vi "Read Digital Voltmeter.vi"(8 "error in (no error)":errorcluster, 11 "VISA resource name":refnum<visa-resource-name>) -> (0 "error out":errorcluster, 1 "5-digit Frequency":dbl, 2 "3-digit DVM":dbl, 3 "VISA resource name out":refnum<visa-resource-name>)   [LabVIEW 2017, in "Agilent 2000 3000 X-Series.lvlib"]
doc: "Returns the displayed value of the digital voltmeter (DVM)."
uses:
  Agilent 2000 3000 X-Series.lvlib
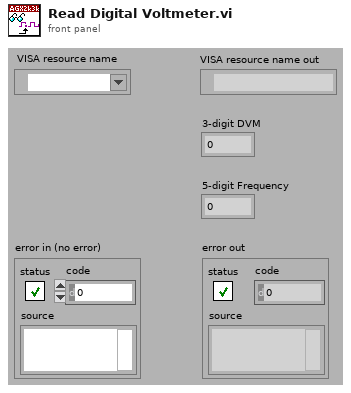
[diagram p1: front panel]
types:
  T1 = typedef "Agilent 2000 3000 X-Series.lvlib/Extended User Data.ctl" = cluster{"X-Series Mode":u16, "Acquisition Type (0: Normal)":i32}
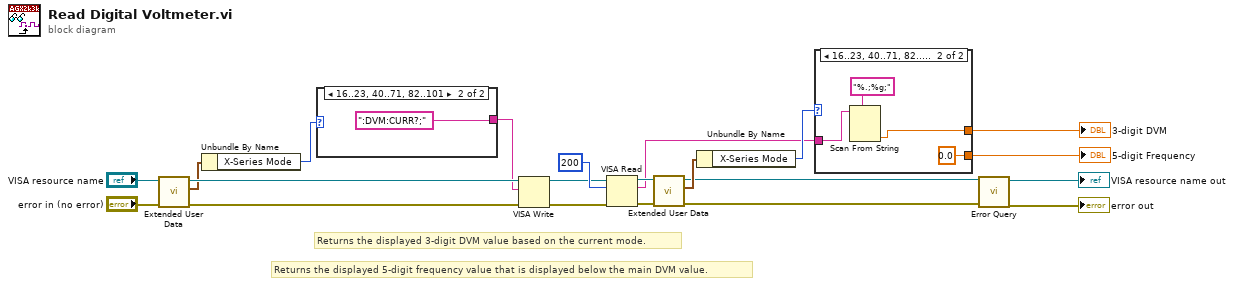
[diagram p0: block diagram]
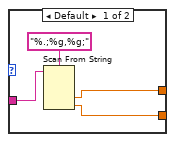
[diagram p2: hidden frame]
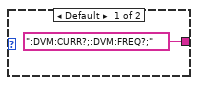
[diagram p3: hidden frame]
diagram:
  # "Returns the displayed 5-digit frequency value that is displayed below the main DVM value."
  # "Returns the displayed 3-digit DVM value based on the current mode."
  n1 = call "Extended User Data.vi"("error in (no error)"="error in (no error)", "VISA resource name in"="VISA resource name") -> ("error out"=w14:errorcluster, "User Data Out"=w9:T1, "VISA resource name out"=w12:refnum<visa-resource-name>)  [unwired: 7 in]
  n2 = Unbundle By Name(w9) -> ("X-Series Mode"=w8:u16)
  n3 = case shown="16..23, 40..71, 82..101" w8 {
    tunnel: [":DVM:CURR?;:DVM:FREQ?;" ":DVM:CURR?;"] -> w10
    frame Default {
    }
    frame 16..23, 40..71, 82..101 {
    }
  }
  n4 = VISA Write(VISA resource name=w12, write buffer=w10, error in (no error)=w14) -> (VISA resource name out=w18:refnum<visa-resource-name>, error out=w17:errorcluster)  [unwired: 1 out]
  n5 = VISA Read(VISA resource name=w18, byte count=u32 200, error in (no error)=w17) -> (VISA resource name out=w6:refnum<visa-resource-name>, read buffer=w3:string, error out=w5:errorcluster)  [unwired: 1 out]
  n6 = call "Extended User Data.vi"("error in (no error)"=w5, "VISA resource name in"=w6) -> ("error out"=w1:errorcluster, "User Data Out"=w7:T1, "VISA resource name out"=w2:refnum<visa-resource-name>)  [unwired: 7 in]
  n7 = Unbundle By Name(w7) -> ("X-Series Mode"=w4:u16)
  n8 = case shown="16..23, 40..71, 82..101" w4 {
    tunnel: [w26 w30] -> w16
    tunnel: [w25 0.0] -> w15
    tunnel: w3 -> [w24 w29]
    frame Default {
      n9 = Scan From String(format string="%.;%g,%g;", input string=w24) -> (output 1=w26:dbl, output 2=w25:dbl)  [unwired: 2 in, 5 out]
    }
    frame 16..23, 40..71, 82..101 {
      n10 = Scan From String(format string="%.;%g;", input string=w29) -> (output 1=w30:dbl)  [unwired: 2 in, 4 out]
    }
  }
  "3-digit DVM" <- w16
  "5-digit Frequency" <- w15
  n11 = call "Error Query.vi"("error in (no error)"=w1, "VISA resource name"=w2) -> ("error out"=→"error out":errorcluster, "VISA resource name out"=→"VISA resource name out":refnum<visa-resource-name>)  [unwired: 8 out]
